vi "rep_cap_init_all.vi"(8 "error in":errorcluster caption="error in (no error)", 9 "Repeated Capabilities":T1[](array[typedef]), 11 "VISA resource name":refnum<visa-resource-name>) -> (0 "error out":errorcluster, 3 "VISA resource name out":refnum<visa-resource-name>)   [LabVIEW 2022 SP3, in "hmp4000_rsidr_core.lvlib"]
uses:
  hmp4000_rsidr_core.lvlib
  type_Input_Format_RepCap.ctl
  _type_Operation_Fgv_RepCap.ctl
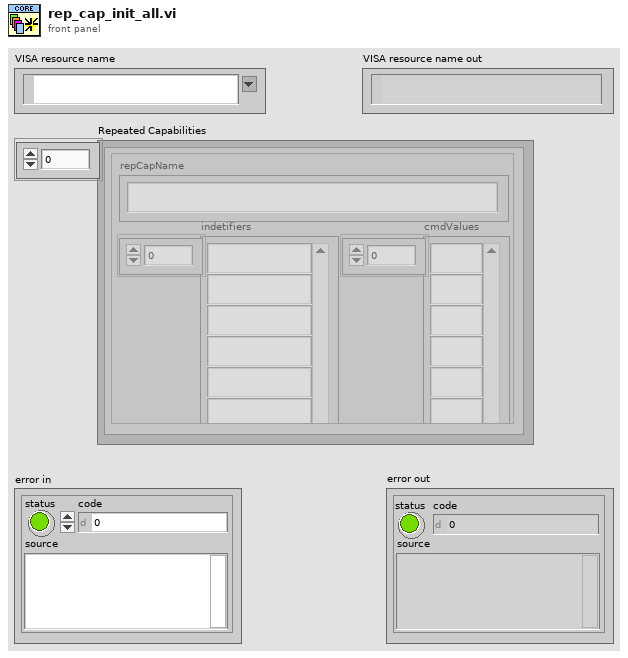
[diagram p1: front panel]
types:
  T1 = typedef "hmp4000_rsidr_core.lvlib/type_Input_Format_RepCap.ctl" = cluster{"repCapName":string, "indetifiers":string[], "cmdValues":string[]}
  T2 = typedef "hmp4000_rsidr_core.lvlib/_type_Operation_Fgv_RepCap.ctl" = enum16{"Initialize", "Get Cmd Value", "Reset Rep Cap", "Add Rep Cap", "Remove Rep Cap", "Get Rep Cap ID range", "Get Count", "Clear", "Find Name from NameID", "Get First NameID"}
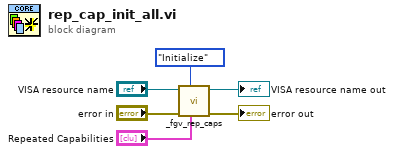
[diagram p0: block diagram]
diagram:
  n1 = call "_fgv_rep_caps.vi"("Repeated Capabilities (empty)"="Repeated Capabilities", "Operation"=_type_Operation_Fgv_RepCap."Initialize", "error in"="error in", "VISA resource name"="VISA resource name") -> ("error out"=→"error out":errorcluster, "VISA resource name out"=→"VISA resource name out":refnum<visa-resource-name>)  [unwired: 4 in, 2 out]
